vi "Simulation Call Statechart (DLL).vi"(4 "operation":T14, 5 "Robot Index":i32, 8 "error in (no error)":errorcluster, 10 "Array Sensors In":T1[](array[typedef]) {"Kobuki Sensors"."Infrared" format="%02x"; "iRobot Sensors"."Infrared" format="%02x"; "accelerometer"."z axis (g)" format="%.3f"; "accelerometer"."y axis (g)" format="%.3f"; "accelerometer"."x axis (g)" format="%.3f"}, 11 "simulator":T15={"configuration"={"maxTime"=5.0, "enableVisualization"=TRUE, "Environment Definition"=path "simulation configuration.ini", "Record Location"=path "Simulation Record.xml", "autograde?"=TRUE, "interactive?"=FALSE, "Feedback Mode"=enum."debug navigation", "Robot State Charts"=[path "C:/Users/blueuser/Desktop/Robo Sim Berkley/cpsgrader-release-0.4/Simulators/EECS149lab/src/LabVIEW/statechart/Simulation Statechart.vi"], "statechart"=path "C:/Users/blueuser/Desktop/Robo Sim Berkley/cpsgrader-release-0.4/Simulators/EECS149lab/src/LabVIEW/statechart/Simulation Statechart.vi"}, "Statechart\ndisplay"=refnum, "first step?"=FALSE, "Robots Simulation Statecharts"=[], "Robots"=[]}) -> (0 "error out":errorcluster, 2 "Array Sensors Out":T1[](array[typedef]) {"Kobuki Sensors"."Infrared" format="%02x"; "iRobot Sensors"."Infrared" format="%02x"; "accelerometer"."z axis (g)" format="%.3f"; "accelerometer"."y axis (g)" format="%.3f"; "accelerometer"."x axis (g)" format="%.3f"}, 3 "simulator":T15={"configuration"={"maxTime"=5.0, "enableVisualization"=TRUE, "Environment Definition"=path "simulation configuration.ini", "Record Location"=path "Simulation Record.xml", "autograde?"=TRUE, "interactive?"=FALSE, "Feedback Mode"=enum."debug navigation", "Robot State Charts"=[path "C:/Users/blueuser/Desktop/Robo Sim Berkley/cpsgrader-release-0.4/Simulators/EECS149lab/src/LabVIEW/statechart/Simulation Statechart.vi"], "statechart"=path "C:/Users/blueuser/Desktop/Robo Sim Berkley/cpsgrader-release-0.4/Simulators/EECS149lab/src/LabVIEW/statechart/Simulation Statechart.vi"}, "Statechart\ndisplay"=refnum, "first step?"=FALSE, "Robots Simulation Statecharts"=[], "Robots"=[]})   [LabVIEW 2014]
uses:
  Simulator.ctl
  CyberSim interface/Simulation Configuration.ctl
  autograder/feedbackMode.ctl
  Multi Bot Code/RobotData.ctl
  <instrlib>/DC Motor Controller/HAIOL/DC Motor Controller.lvclass
  Simulation Call Statechart Operation.ctl
  shared/Sensors.ctl
  iRobot/Sensor/Accelerometer.ctl
  iRobot/Sensor/Sensor Group 6.ctl
  iRobot/Sensor/Bumps + Wheel Drops.ctl
  iRobot/Sensor/Buttons.ctl
  iRobot/Sensor/Charging State.ctl
  iRobot/Sensor/Charging Sources Available.ctl
  iRobot/Sensor/OI Mode.ctl
  iRobot/Sensor/Cargo Bay Digital Inputs.ctl
  iRobot/Sensor/Low-Side Driver + Wheel Overcurrent.ctl
  Kobuki/KobukiSensors.ctl
  Kobuki/Kobuki Bumps and WheelDrops.ctl
  Kobuki/Kobuki Buttons.ctl
panel:
  # "Electrical: charging, battery, OI mode"
  # "Sensors: bump, cliff, button, wheel drop, wall, virtual wall"
  # "Motion: distance, angle, requested velocity"
  # "Cargo Bay: I/O, overcurrent, infrared"
  # "Song"
  # "Electrical: charging, battery, OI mode"
  # "Sensors: bump, cliff, button, wheel drop, wall, virtual wall"
  # "Motion: distance, angle, requested velocity"
  # "Cargo Bay: I/O, overcurrent, infrared"
  # "Song"
  # "Electrical: charging, battery, OI mode"
  # "Sensors: bump, cliff, button, wheel drop, wall, virtual wall"
  # "Motion: distance, angle, requested velocity"
  # "Cargo Bay: I/O, overcurrent, infrared"
  # "Song"
  # "Electrical: charging, battery, OI mode"
  # "Sensors: bump, cliff, button, wheel drop, wall, virtual wall"
  # "Motion: distance, angle, requested velocity"
  # "Cargo Bay: I/O, overcurrent, infrared"
  # "Song"
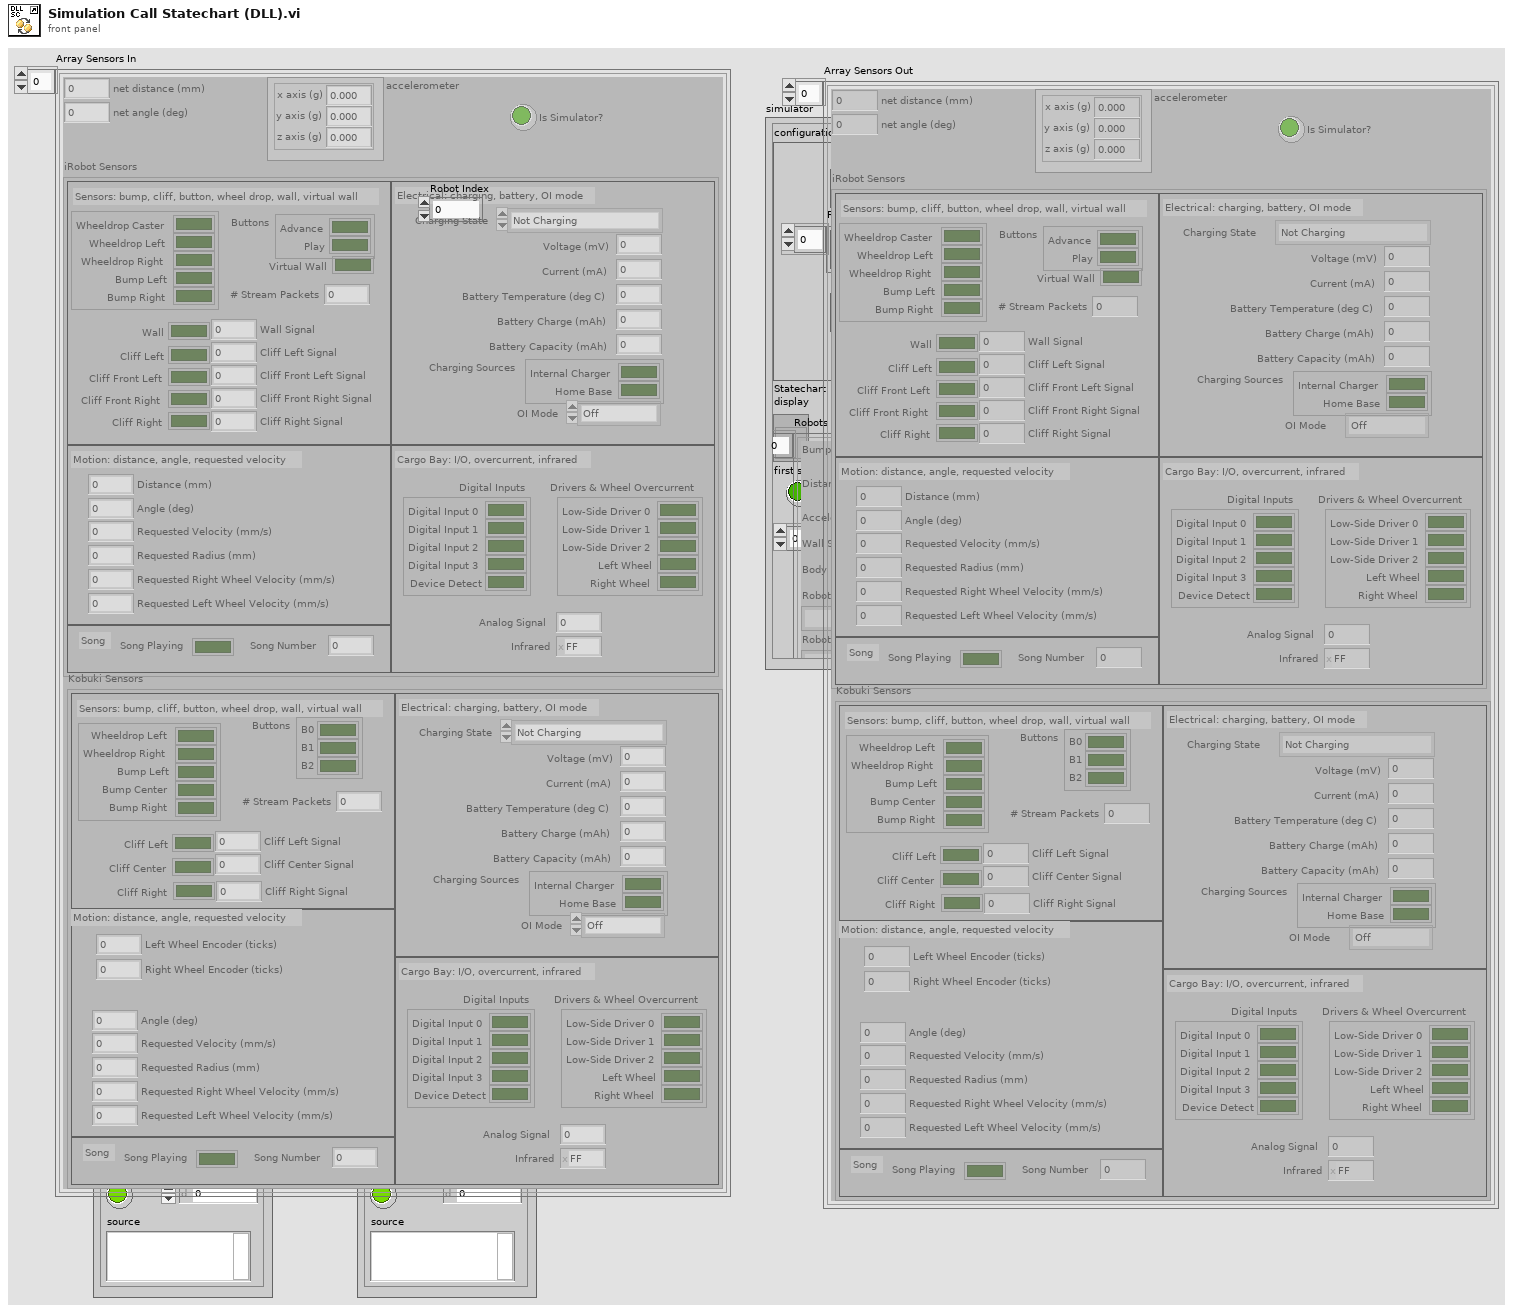
[diagram p1: front panel]
types:
  T1 = typedef "Sensors.ctl" = cluster{"net distance (mm)":i32, "net angle (deg)":i32, "accelerometer":T2, "iRobot Sensors":T3, "Is Simulator?":bool, "Kobuki Sensors":T11}
  T2 = typedef "Accelerometer.ctl" = cluster{"x axis (g)":dbl, "y axis (g)":dbl, "z axis (g)":dbl}
  T3 = typedef "Sensor Group 6.ctl" = cluster{"Bumps + Wheel Drops":T4, "Wall":bool, "Cliff Left":bool, "Cliff Front Left":bool, "Cliff Front Right":bool, "Cliff Right":bool, "Wall Signal":u16, "Cliff Left Signal":u16, "Cliff Front Left Signal":u16, "Cliff Front Right Signal":u16, "Cliff Right Signal":u16, "Buttons":T5, "Virtual Wall":bool, "# Stream Packets":u8, "Requested Velocity (mm/s)":i16, "Requested Radius (mm)":i16, "Requested Right Wheel Velocity (mm/s)":i16, "Requested Left Wheel Velocity (mm/s)":i16, "Distance (mm)":i32, "Angle (deg)":i32, "Song Playing":bool, "Song Number":u8, "Charging State":T6, "Voltage (mV)":u16, "Current (mA)":i16, "Battery Temperature (deg C)":i8, "Battery Charge (mAh)":u16, "Battery Capacity (mAh)":u16, "Charging Sources":T7, "OI Mode":T8, "Digital Inputs":T9, "Drivers & Wheel Overcurrent":T10, "Analog Signal":u16, "Infrared":u8}
  T4 = typedef "Bumps + Wheel Drops.ctl" = cluster{"Wheeldrop Caster":bool, "Wheeldrop Left":bool, "Wheeldrop Right":bool, "Bump Left":bool, "Bump Right":bool}
  T5 = typedef "Buttons.ctl" = cluster{"Advance":bool, "Play":bool}
  T6 = typedef "Charging State.ctl" = enum16{"Not Charging", "Reconditioning Charging", "Full Charging", "Trickle Charging", "Waiting", "Charging Fault Condition"}
  T7 = typedef "Charging Sources Available.ctl" = cluster{"Internal Charger":bool, "Home Base":bool}
  T8 = typedef "OI Mode.ctl" = enum16{"Off", "Passive", "Safe", "Full"}
  T9 = typedef "Cargo Bay Digital Inputs.ctl" = cluster{"Digital Input 0":bool, "Digital Input 1":bool, "Digital Input 2":bool, "Digital Input 3":bool, "Device Detect":bool}
  T10 = typedef "Low-Side Driver + Wheel Overcurrent.ctl" = cluster{"Low-Side Driver 0":bool, "Low-Side Driver 1":bool, "Low-Side Driver 2":bool, "Left Wheel":bool, "Right Wheel":bool}
  T11 = typedef "KobukiSensors.ctl" = cluster{"Bumps + Wheel Drops":T12, "Cliff Left":bool, "Cliff Center":bool, "Cliff Right":bool, "Cliff Left Signal":u16, "Cliff Center Signal":u16, "Cliff Right Signal":u16, "Buttons":T13, "# Stream Packets":u8, "Requested Velocity (mm/s)":i16, "Requested Radius (mm)":i16, "Requested Right Wheel Velocity (mm/s)":i16, "Requested Left Wheel Velocity (mm/s)":i16, "Left Wheel Encoder (ticks)":i16, "Angle (deg)":i32, "Song Playing":bool, "Song Number":u8, "Charging State":T6, "Voltage (mV)":u16, "Current (mA)":i16, "Battery Temperature (deg C)":i8, "Battery Charge (mAh)":u16, "Battery Capacity (mAh)":u16, "Charging Sources":T7, "OI Mode":T8, "Digital Inputs":T9, "Drivers & Wheel Overcurrent":T10, "Analog Signal":u16, "Infrared":u8, "Right Wheel Encoder (ticks) ":i16}
  T12 = typedef "Kobuki Bumps and WheelDrops.ctl" = cluster{"Wheeldrop Left":bool, "Wheeldrop Right":bool, "Bump Left":bool, "Bump Center":bool, "Bump Right":bool}
  T13 = typedef "Kobuki Buttons.ctl" = cluster{"B0":bool, "B1":bool, "B2":bool}
  T14 = typedef "Simulation Call Statechart Operation.ctl" = enum16{"Initialize", "Call Statechart", "Finalize"}
  T15 = typedef "Simulator.ctl" = cluster{"configuration":T16, "Statechart\ndisplay":refnum<vi>, "first step?":bool, "Robots Simulation Statecharts":path[], "Robots":T18[]}
  T16 = typedef "Simulation Configuration.ctl" = cluster{"maxTime":sgl, "enableVisualization":bool, "Environment Definition":path, "Record Location":path, "autograde?":bool, "interactive?":bool, "Feedback Mode":T17, "Robot State Charts":path[], "statechart":path}
  T17 = typedef "feedbackMode.ctl" = enum32{"debug navigation", "debug hill climb", "autograde navigation", "autograde hill climb"}
  T18 = typedef "RobotData.ctl" = cluster{"Bump Sensors":refnum<k20>[], "Distance Sensors":refnum<k20>[], "Accelerometer":refnum<k20>, "Wall Sensor":refnum<k20>, "Body":refnum<k20>, "RobotID":string, "RobotType":string, "Left Motor":refnum<class "DC Motor Controller.lvclass">, "Right Motor":refnum<class "DC Motor Controller.lvclass">}
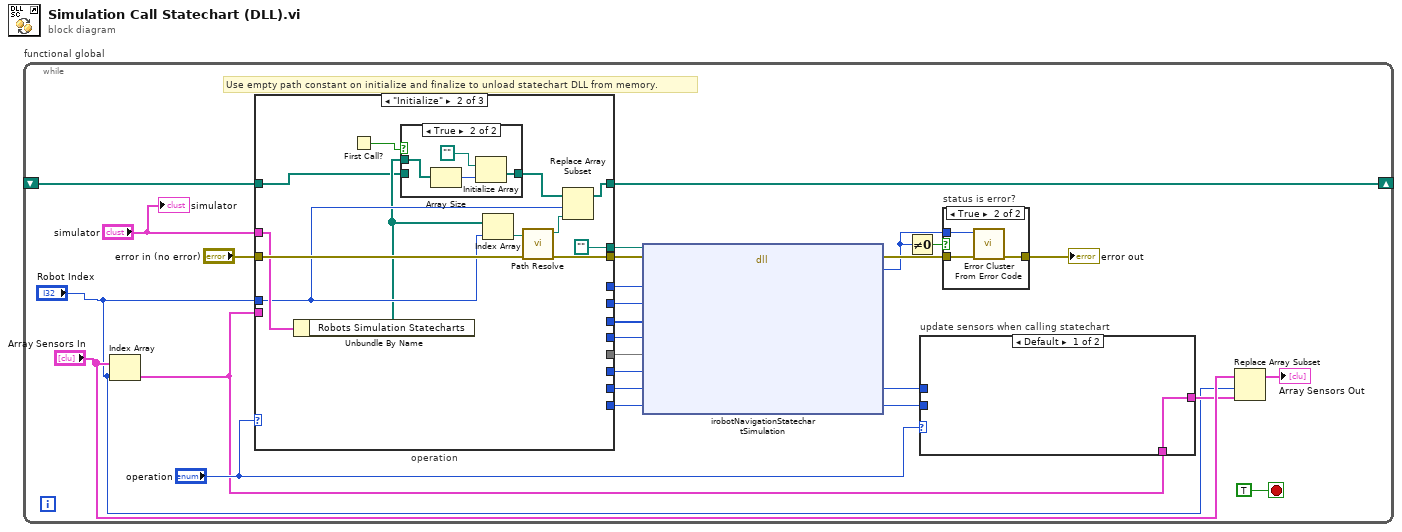
[diagram p0: block diagram]
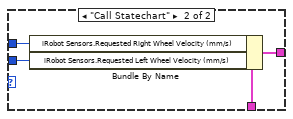
[diagram p2: hidden frame]
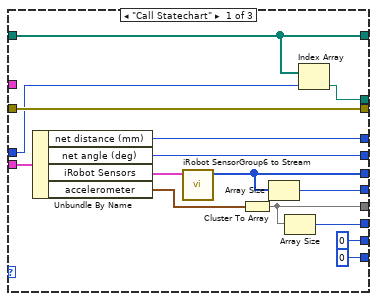
[diagram p4: hidden frame]
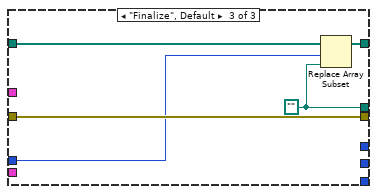
[diagram p6: hidden frame]
diagram:
  n1 = while "functional global" {
    shift-right: [w7] -> _
    shift-left: _ -> [w6]
    stop <- TRUE stop-if-true
    # "Use empty path constant on initialize and finalize to unload statechart DLL from memory."
    n2 = Index Array(array="Array Sensors In", index="Robot Index") -> (element=w5:T1)
    n3 = case "operation" shown="\"Initialize\"" "operation" {
      tunnel: "error in (no error)" -> [w51 w63 w73]
      tunnel: [w51 w62 w73] -> w27
      tunnel: [w39 path "" w70] -> w26
      tunnel: [w38 w58 w71] -> w7
      tunnel: w6 -> [w38 w54 w72]
      tunnel: [w48 _ _] -> w24
      tunnel: [w47 _ _] -> w23
      tunnel: [w46 _ _] -> w22
      tunnel: [w45 _ _] -> w21
      tunnel: [w44 _ _] -> w20
      tunnel: [w43 _ _] -> w19
      tunnel: [i16 0 ("rightWheelSpeed") _ _] -> w18
      tunnel: [i16 0 ("rightWheelSpeed") _ _] -> w17
      tunnel: w5 -> [w40 _ _]
      tunnel: "simulator" -> [_ w60 _]
      tunnel: "Robot Index" -> [w37 w56 w69]
      frame "Call Statechart" {
        n4 = Unbundle By Name(w40) -> ("net distance (mm)"=w48:i32, "net angle (deg)"=w47:i32, "iRobot Sensors"=w49:T3, "accelerometer"=w50:T2)
        n5 = call "iRobot SensorGroup6 to Stream.vi"("iRobot Sensor Group 6"=w49) -> ("stream"=w46:u8[])  [unwired: 9 in, 1 out]
        n6 = Cluster To Array(cluster=w50) -> (array=w44:dbl[])
        n7 = Array Size(array=w46) -> (size(s)=w45:i32)
        n8 = Array Size(array=w44) -> (size(s)=w43:i32)
        n9 = Index Array(array=w38, index=w37) -> (element=w39:path)
      }
      frame "Initialize" {
        n10 = Unbundle By Name(w60) -> ("Robots Simulation Statecharts"=w55:path[])
        n11 = First Call?() -> (First Call?: T/F=w52:bool)
        n12 = case shown="True" w52 {
          tunnel: w54 -> [w64 _]
          tunnel: [w64 w66] -> w53
          tunnel: w55 -> [_ w67]
          frame False {
          }
          frame True {
            n13 = Array Size(array=w67) -> (size(s)=w68:i32)
            n14 = Initialize Array(path "", w68) -> (w66:path[])
          }
        }
        n15 = Index Array(array=w55, index=w56) -> (element=w59:path)
        n16 = call "Path Resolve.vi"("Error In"=w63, "absolute or relative path"=w59) -> ("Error Out"=w62:errorcluster, "resolved path"=w57:path)  [unwired: 8 in]
        n17 = Replace Array Subset(array=w53, new element=w57, index=w56) -> (w58:path[])
      }
      frame "Finalize", Default {
        w70 = path ""
        n18 = Replace Array Subset(array=w72, new element=w70, index=w69) -> (w71:path[])
      }
    }
    n19 = dll-call lib="D:/Users/jjensen/workspace/Simulated iRobot Navigation/Release/libSimulated iRobot Navigation.dll" fn="irobotNavigationStatechartSimulation"(path in=w26, error in=w27, "netDistance"=w24, "netAngle"=w23, "sensorStream"=w22, "sensorStreamSize"=w21, "accelAxes"=w20, "accelAxesSize"=w19, "rightWheelSpeed"=w18, "leftWheelSpeed"=w17) -> (error out=w13:errorcluster, "status"=w12:i32, "rightWheelSpeed"=w10:i16, "leftWheelSpeed"=w9:i16)  [unwired: 7 in, 1 out]
    n20 = Not Equal To 0?(x=w12) -> (x != 0?=w15:bool)
    n21 = case "update sensors when calling statechart" shown="Default" "operation" {
      tunnel: w10 -> [_ w32]
      tunnel: w9 -> [_ w31]
      tunnel: w5 -> [w28 w30]
      tunnel: [w28 w29] -> w3
      frame Default {
      }
      frame "Call Statechart" {
        n22 = Bundle By Name(cluster=w30, "iRobot Sensors.Requested Right Wheel Velocity (mm/s)"=w32, "iRobot Sensors.Requested Left Wheel Velocity (mm/s)"=w31) -> (w29:T1)
      }
    }
    n23 = case "status is error?" shown="True" w15 {
      tunnel: w12 -> [_ w36]
      tunnel: w13 -> [w33 w35]
      tunnel: [w33 w34] -> w14
      frame False {
      }
      frame True {
        n24 = call <vilib>:"Error Cluster From Error Code.vi"("error in (no error)"=w35, "error code (0)"=w36) -> ("error out"=w34:errorcluster)  [unwired: 7 in]
      }
    }
    "error out" <- w14
    n25 = Replace Array Subset(array="Array Sensors In", new element=w3, index="Robot Index") -> (→"Array Sensors Out":T1[])
    "simulator" <- "simulator"
  }
